vi "Enqueue one state to model.vi"(6 "Priority? (F)":bool, 8 "error in (no error)":errorcluster, 9 "Following state if error":string, 10 "Enqueued data":variant, 11 "Enqueued state":string) -> (0 "error out":errorcluster)   [LabVIEW 2018]
doc: "Enqueued State: Case-insensitive string that names the case that this entry in the queue will run.\nEnqueued Data: Variant containing any data needed by the case in the queue.\n\nOptional inputs:\nFollowing state if error: If left blank, any error in the controller loop will clear the controller queue and send the error as data to the default \"Error Handler\" state. If filled in, instead of going to the error state next it will go to the specified state, with the error enqueued as the \"Data\" variant.\nPriority: If True, uses the \"Enqueue at opposite end\" node to move this next state to the front of the line. Use with caution, as this could disrupt sequenced operations."
uses:
  Model queue data.ctl
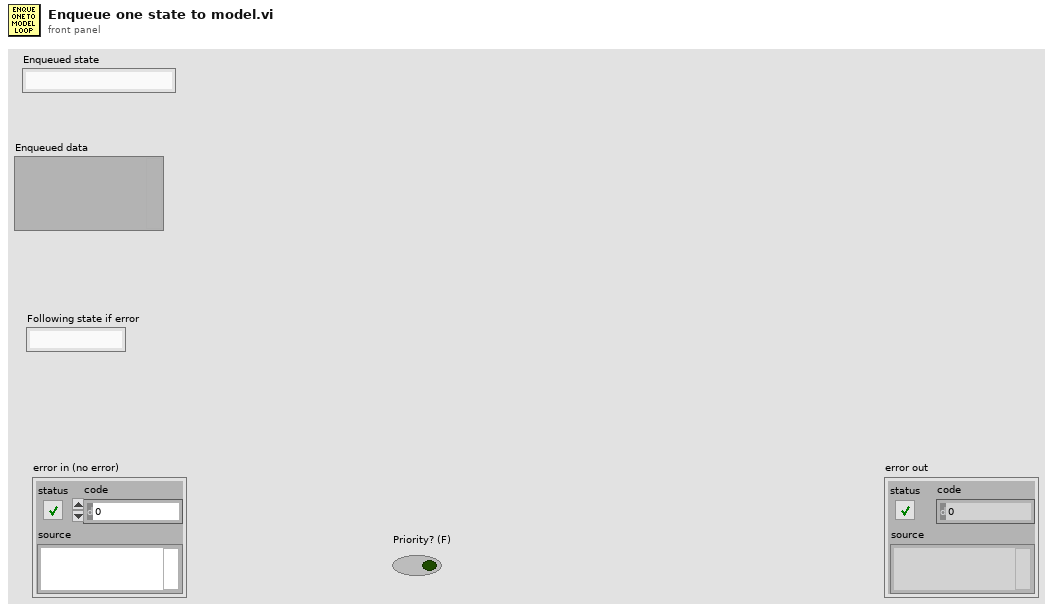
[diagram p1: front panel]
types:
  T1 = typedef "Model queue data.ctl" = cluster{"State":string, "Data":variant, "Next state if error":string}
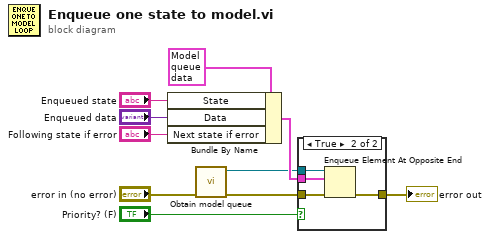
[diagram p0: block diagram]
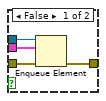
[diagram p2: hidden frame]
diagram:
  n1 = Bundle By Name(cluster=T1 {"State"="", "Data"=variant, "Next state if error"=""} ("element"), "State"="Enqueued state", "Data"="Enqueued data", "Next state if error"="Following state if error") -> (w7:T1)
  n2 = call "Obtain model queue.vi"("error in (no error)"="error in (no error)") -> ("error out"=w9:errorcluster, "Model loop queue"=w1:refnum<queue>)  [unwired: 9 in]
  n3 = case shown="True" "Priority? (F)" {
    tunnel: w9 -> [w14 w18]
    tunnel: w7 -> [w13 w17]
    tunnel: [w12 w16] -> w6
    tunnel: w1 -> [w11 w15]
    frame False {
      n4 = Enqueue Element(queue=w11, element=w13, error in (no error)=w14) -> (error out=w12:errorcluster)  [unwired: 1 in, 2 out]
    }
    frame True {
      n5 = Enqueue Element At Opposite End(queue=w15, element=w17, error in (no error)=w18) -> (error out=w16:errorcluster)  [unwired: 1 in, 2 out]
    }
  }
  "error out" <- w6
